vi "Game Controller Open.vi"(8 "error in":errorcluster, 11 "Device Index":i32 format="%.0x") -> (0 "error out":errorcluster, 3 "Game Controller Pointer":u32 format="%.0x")   [LabVIEW 2014, in "LibSDL2.lvlib"]
uses:
  LibSDL2.lvlib
  DLL/SDL2.dll
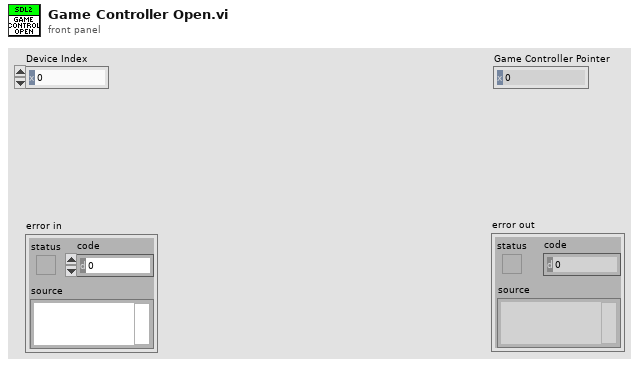
[diagram p1: front panel]
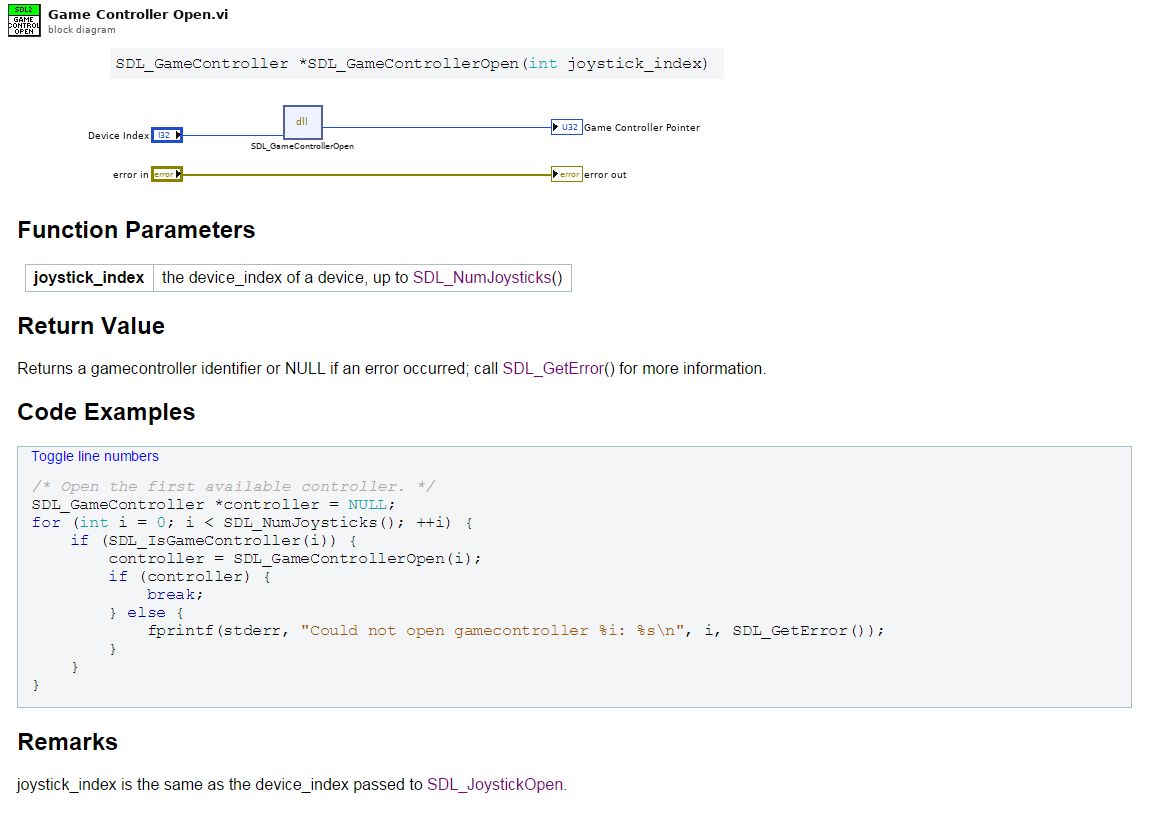
[diagram p0: block diagram]
diagram:
  n1 = dll-call lib="C:/dev/PGS/LabSDL2/Source/LibSDL2 Wrapper/DLL/SDL2.dll" fn="SDL_GameControllerOpen"("device_index"="Device Index") -> ("joystick pointer"=→"Game Controller Pointer":u32)  [unwired: 4 in, 2 out]
  "error out" <- "error in"
